vi "problem3.vi"() -> ()   [LabVIEW 2020]
panel:
  out "Boolean":bool
  in  "B":bool
  in  "A":bool
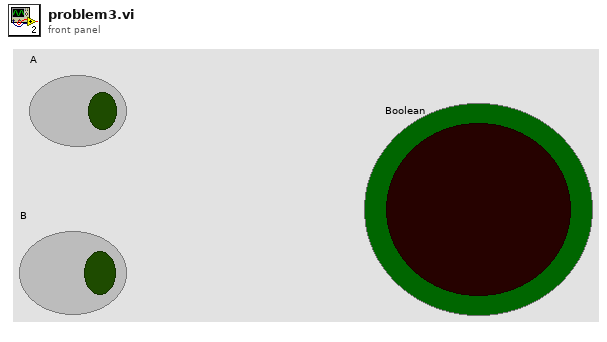
[diagram p1: front panel]
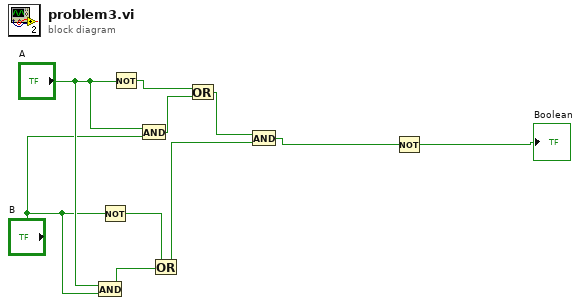
[diagram p0: block diagram]
diagram:
  n1 = And(x="A", y="B") -> (x .and. y?=w5:bool)
  n2 = Not(x="B") -> (.not. x?=w4:bool)
  n3 = Not(x="A") -> (.not. x?=w10:bool)
  n4 = And(x="A", y="B") -> (x .and. y?=w9:bool)
  n5 = Or(x=w4, y=w5) -> (x .or. y?=w3:bool)
  n6 = Or(x=w10, y=w9) -> (x .or. y?=w8:bool)
  n7 = And(x=w8, y=w3) -> (x .and. y?=w2:bool)
  n8 = Not(x=w2) -> (.not. x?=→"Boolean":bool)
